vi "Select Group.vi"(8 "error in (no error)":errorcluster, 10 "Group (Empty = none)":string, 11 "Historian Charting Manager in":refnum<class "Historian Charting Manager.lvclass">) -> (0 "error out":errorcluster, 3 "Historian Charting Manager out":refnum<class "Historian Charting Manager.lvclass">)   [LabVIEW 2020, in "VolatusGUI.lvlib" / "Historian Charting Manager.lvclass"]
uses:
  Historian Charting Manager.lvclass
  Historian Charting Manager.lvclass/Historian Charting Manager.ctl
  X-Axis Type.ctl
  Scale.ctl
  Plot Config.ctl
  Plot Group Config.ctl
  Select Plot Group Data.ctl
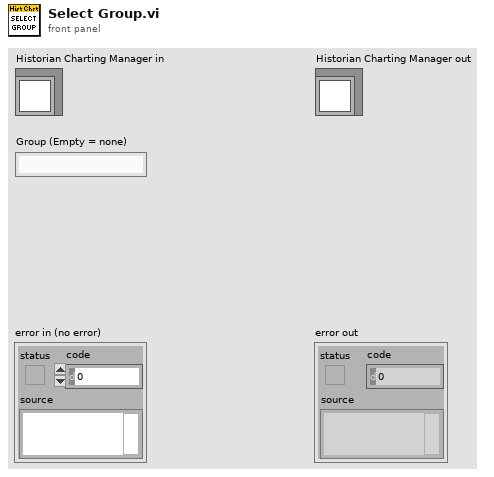
[diagram p1: front panel]
types:
  T1 = typedef "VolatusGUI.lvlib/Historian Charting Manager.lvclass/Plot Group Config.ctl" = cluster{"Name":string, "X-Axis Type":T2, "X-Axis Channel":string, "Plots":T3[], "Lock Now":bool, "Time":string}
  T2 = typedef "VolatusGUI.lvlib/Historian Charting Manager.lvclass/X-Axis Type.ctl" = enum16{"Time", "Channel"}
  T3 = typedef "VolatusGUI.lvlib/Historian Charting Manager.lvclass/Plot Config.ctl" = cluster{"Channel":string, "Visible":bool, "Color":u32, "Scale":T4}
  T4 = typedef "VolatusGUI.lvlib/Historian Charting Manager.lvclass/Scale.ctl" = enum16{"Left", "Right"}
  T5 = typedef "VolatusGUI.lvlib/Historian Charting Manager.lvclass/Chart Registration.ctl" = cluster{"Chart Num":i32, "PluginGUI":refnum<class "MessageQ.lvclass">, "Select Plot Group":refnum<user-event>}
  T6 = typedef "VolatusGUI.lvlib/Historian Charting Manager.lvclass/Select Plot Group Data.ctl" = cluster{"Chart Num":i32, "Plots Config":T1}
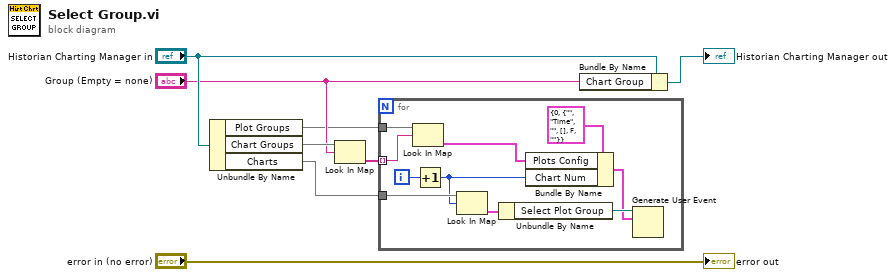
[diagram p0: block diagram]
diagram:
  n1 = Unbundle By Name("Historian Charting Manager in") -> ("Plot Groups"=w2:map{string, T1}, "Chart Groups"=w5:map{string, string[]}, "Charts"=w1:map{i32, T5})
  n2 = Look In Map(map=w5, key="Group (Empty = none)") -> (value=w3:string[])  [unwired: 1 in, 1 out]
  n3 = for {
    tunnel: w3 -> [w13] mode=indexing
    tunnel: w2 -> [w14]
    tunnel: w1 -> [w17]
    i -> [w18]
    n4 = Look In Map(map=w14, key=w13) -> (value=w10:T1)  [unwired: 1 in, 1 out]
    n5 = Increment(x=w18) -> (x+1=w9:i32)
    n6 = Look In Map(map=w17, key=w9) -> (value=w16:T5)  [unwired: 1 in, 1 out]
    n7 = Unbundle By Name(w16) -> ("Select Plot Group"=w15:refnum<user-event>)
    n8 = Bundle By Name(cluster=T6 {"Chart Num"=0, "Plots Config"={"Name"="", "X-Axis Type"=enum."Time", "X-Axis Channel"="", "Plots"=[], "Lock Now"=FALSE, "Time"=""}} ("event data"), "Plots Config"=w10, "Chart Num"=w9) -> (w11:T6)
    n9 = Generate User Event(user event=w15, event data cluster=w11) -> ()  [unwired: 2 in, 2 out]
  }
  n10 = Bundle By Name(cluster="Historian Charting Manager in", "Chart Group"="Group (Empty = none)") -> (→"Historian Charting Manager out":refnum<class "Historian Charting Manager.lvclass">)
  "error out" <- "error in (no error)"
